vi "TQFLSHdll_d.vi"(5 "dll_path_in":path, 8 "error in (no error)":errorcluster, 9 "Component Molar Fractions":dbl[](array[numeric])=[1.0, 0.0, 0.0, 0.0, 0.0, 0.0, 0.0, 0.0, 0.0, 0.0, 0.0, 0.0, 0.0, 0.0, 0.0, 0.0, 0.0, 0.0, 0.0, 0.0], 10 "Q":dbl=1.0 min=0.0 max=1.0 step=0.05, 11 "T":dbl=30.0) -> (0 "error out":errorcluster, 3 "tqdataout":dbl[](array[numeric]), 4 "dll_path_out":path)   [LabVIEW 2017]
doc: "Please feel free to contact me if you have any questions .\nMy mail:ken_pop@tom.com yan.ding@jci.com"
panel:
  out "x":dbl[](array[numeric])
  out "d":dbl
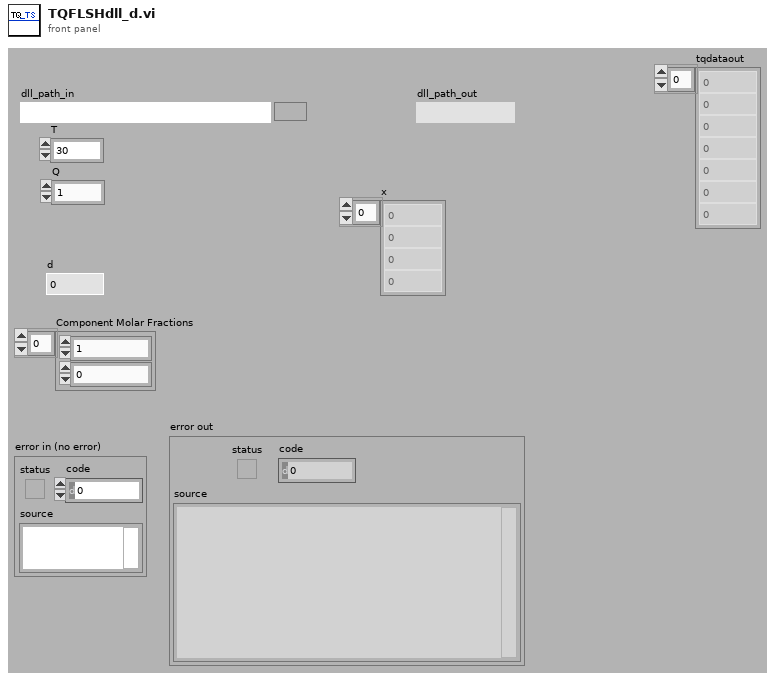
[diagram p1: front panel]
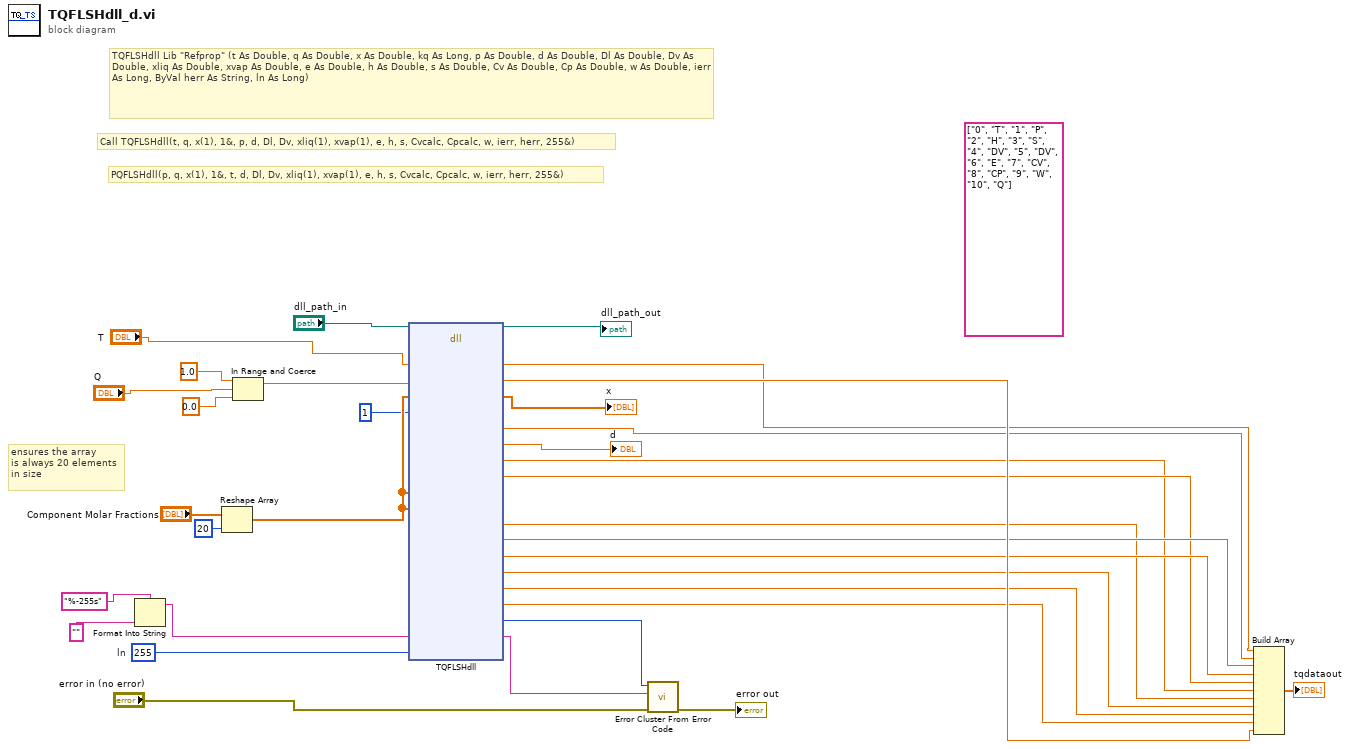
[diagram p0: block diagram]
diagram:
  (unwired) string[][] [["0", "T"], ["1", "P"], ["2", "H"], ["3", "S"], ["4", "DV"], ["5", "DV"], ["6", "E"], ["7", "CV"], ["8", "CP"], ["9", "W"], ["10", "Q"]] ("数组")
  w25 = 255  # ln
  # "Call TQFLSHdll(t, q, x(1), 1&, p, d, Dl, Dv, xliq(1), xvap(1), e, h, s, Cvcalc, Cpcalc, w, ierr, herr, 255&)"
  # "TQFLSHdll Lib \"Refprop\" (t As Double, q As Double, x As Double, kq As Long, p As Double, d As Double, Dl As Double, Dv As Double, xliq As Double, xvap As Double, e As Double, h As Double, s As Double, Cv As Double, Cp As Double, w As Double, ierr As Long, ByVal herr As String, ln As Long)"
  # "PQFLSHdll(p, q, x(1), 1&, t, d, Dl, Dv, xliq(1), xvap(1), e, h, s, Cvcalc, Cpcalc, w, ierr, herr, 255&)"
  # "ensures the array\nis always 20 elements\nin size"
  n1 = Format Into String(format string="%-255s", "") -> (resulting string=w24:string)  [unwired: 2 in, 1 out]
  n2 = Reshape Array("Component Molar Fractions", 20 ("dimension size")) -> (w21:dbl[])
  n3 = In Range and Coerce(upper limit=1.0 ("上限"), x="Q", lower limit=0.0 ("下限")) -> (coerced(x)=w13:dbl)  [unwired: 1 out]
  n4 = dll-call lib="refprop.DLL" fn="TQFLSHdll"(path in="dll_path_in", "t"="T", "q"=w13, "x"=w21, "1&"=1, "xliq"=w21, "xvap"=w21, "herr"=w24, "ln"=w25) -> (path out=→"dll_path_out":path, "t"=w2:dbl, "q"=w11:dbl, "x"=→"x":dbl[], "p"=w1:dbl, "d"=→"d":dbl, "Dl"=w7:dbl, "Dv"=w8:dbl, "e"=w6:dbl, "h"=w10:dbl, "s"=w9:dbl, "cv"=w5:dbl, "cp"=w4:dbl, "w"=w3:dbl, "ierr"=w26:i32, "herr"=w27:string)  [unwired: 18 in, 1 out]
  n5 = call <vilib>:"Error Cluster From Error Code.vi"("error in (no error)"="error in (no error)", "error message (\"\")"=w27, "error code (0)"=w26) -> ("error out"=→"error out":errorcluster)  [unwired: 6 in]
  n6 = Build Array(w2, w1, w10, w9, w8, w7, w6, w5, w4, w3, w11) -> (→"tqdataout":dbl[])
